vi "BESSY Event Test.vi"() -> ()   [LabVIEW 2011]
panel:
  out "Set Point":dbl[](array[numeric])
  in  "stop":bool
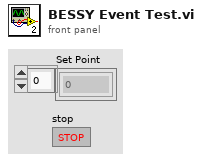
[diagram p1: front panel]
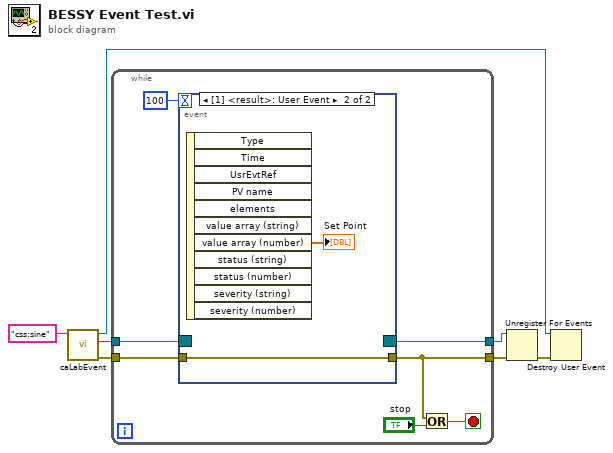
[diagram p0: block diagram]
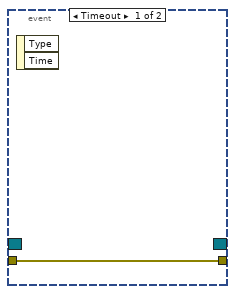
[diagram p2: hidden frame]
diagram:
  n1 = call <userlib>:"caLabEvent.vi"("PV name"="css:sine") -> ("error out"=w5:errorcluster, "refnum"=w7:refnum<event-registration>, "event"=w1:refnum<user-event>)  [unwired: 8 in]
  n2 = while {
    tunnel: w7 -> [w13]
    tunnel: w5 -> [w10]
    tunnel: [w9] -> w3
    tunnel: [w8] -> w2
    stop <- w11 stop-if-true
    n3 = event shown="[1] <result>: User Event" {
      selector: w13 -> [_ _]
      dyn-events: [_ _] -> w8
      timeout: 100 -> [_ _]
      tunnel: w10 -> [w15 w16]
      tunnel: [w15 w16] -> w9
      event Timeout {
        n4 = event-data() -> ()  [unwired: 1 in, 2 out]
      }
      event User Event {
        n5 = event-data() -> ("value array (number)"=→"Set Point":dbl[])  [unwired: 1 in, 10 out]
      }
    }
    n6 = Or(x=w9, y="stop") -> (x .or. y?=w11:bool)
  }
  n7 = Unregister For Events(event registration refnum=w2, error in=w3) -> (error out=w4:errorcluster)
  n8 = Destroy User Event(user event=w1, error in=w4) -> ()  [unwired: 1 out]
